vi "Add Tx Label.vi"(6 "transfer type":T2, 8 "error in":errorcluster, 9 "SDI value":T3=-1 items=["All"=-1, "0 (b00)"=0, "1 (b01)"=1, "2 (b10)"=2, "3 (b11)"=3], 10 "label value":u32, 11 "port ref":T1 format="%.0x") -> (0 "error out":errorcluster, 2 "label ref":T1 format="%.0x", 3 "port ref out":T1 format="%.0x")   [LabVIEW 2020, in "Ballard ARINC 429 Scripting.lvlib"]
uses:
  Ballard ARINC 429 Scripting.lvlib
  Shared/SDI.ctl
  Shared/Transfer Type.ctl
  <vilib>/NI VeriStand/Custom Device API/Custom Device Item Ref.ctl
  Shared/Label Properties.ctl
  Shared/Label.ctl
  <vilib>/NI VeriStand/Custom Device API/Custom Device Channel.ctl
  <vilib>/NI VeriStand/Custom Device API/Custom Device Channel Type.ctl
  Constants.vi
  <vilib>/NI VeriStand/Custom Device API/Custom Device API.lvlib
  ARINC 429/ARINC 429 Scripting.lvlib
  Import/ARINC 429 Import.lvlib
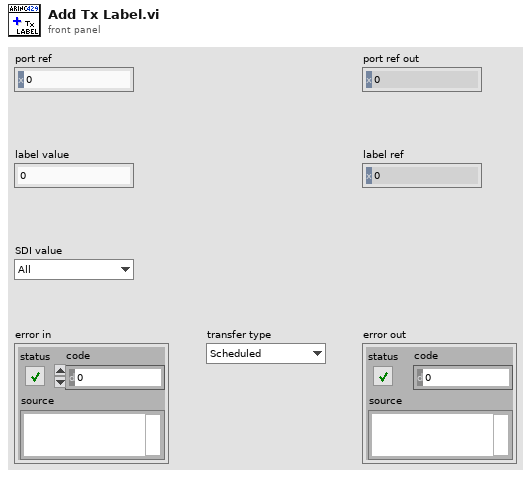
[diagram p1: front panel]
types:
  T1 = typedef "Custom Device API.lvlib/Custom Device Item Ref.ctl" = u64
  T2 = typedef "Transfer Type.ctl" = enum16{"Scheduled", "Acyclic", "Block", "Strobe"}
  T3 = typedef "SDI.ctl" = i32
  T4 = typedef "Direction.ctl" = enum16{"Rx", "Tx"}
  T5 = typedef "Custom Device API.lvlib/Custom Device Channel.ctl" = cluster{"Type":T6, "Units":string, "Default Value":dbl, "Faultable":bool, "Scalable":bool}
  T6 = typedef "Custom Device API.lvlib/Custom Device Channel Type.ctl" = enum16{"Input", "Output"}
  T7 = typedef "Label Properties.ctl" = cluster{"label (Dec)":T8, "SDI value":u8, "SDI enabled":bool}
  T8 = typedef "Label.ctl" = u8
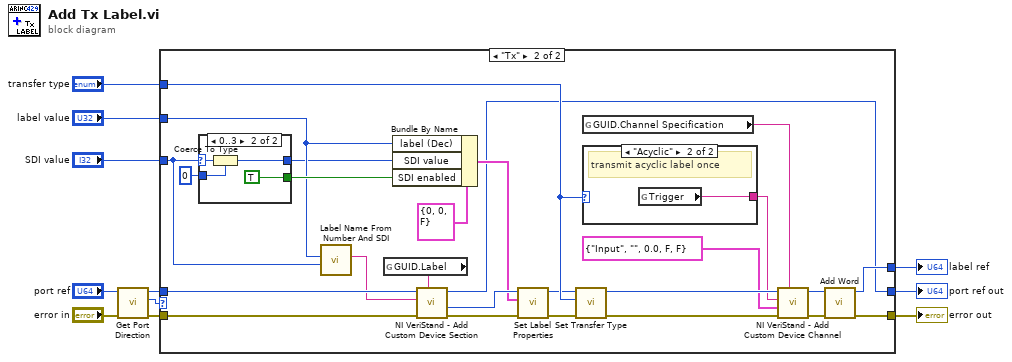
[diagram p0: block diagram]
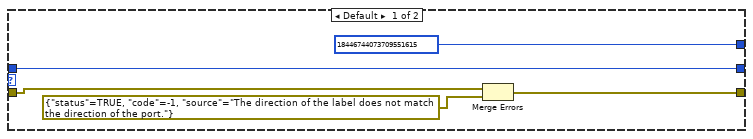
[diagram p2: hidden frame]
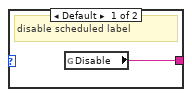
[diagram p3: hidden frame]
diagram:
  n1 = call "Get Port Direction.vi"("error in"="error in", "port ref in"="port ref") -> ("error out"=w7:errorcluster, "direction"=w1:T4, "port ref out"=w8:T1)  [unwired: 7 in]
  n2 = case shown="\"Tx\"" w1 {
    tunnel: [w13 w34] -> w11
    tunnel: w8 -> [w16 w31]
    tunnel: w7 -> [w14 w30]
    tunnel: [T1 18446744073709551615 ("label ref out") w27] -> w6
    tunnel: [w16 w17] -> w5
    tunnel: "transfer type" -> [_ w26]
    tunnel: "label value" -> [_ w23]
    tunnel: "SDI value" -> [_ w21]
    frame Default {
      n3 = Merge Errors(w14, errorcluster {"status"=TRUE, "code"=-1, "source"="The direction of the label does not match the direction of the port."} ("error in")) -> (w13:errorcluster)
    }
    frame "Tx" {
      n4 = case shown="0..3" w21 {
        selector: w21 -> [_ w49]
        tunnel: [w45 w46] -> w22
        tunnel: u8 0 ("SDI value") -> [w45 w48]
        tunnel: [_ TRUE] -> w28
        frame Default {
        }
        frame 0..3 {
          n5 = Coerce To Type(0:w49, 1:w48) -> (2:w46:u8)
        }
      }
      n6 = call "Label Name From Number And SDI.vi"("SDI value"=w21, "label (Dec)"=w23) -> ("label name"=w24:string)  [unwired: 9 in]
      n7 = global read "Constants.vi" "GUID.Label"() -> (w35:string)
      n8 = Bundle By Name(cluster=T7 {"label (Dec)"=0, "SDI value"=0, "SDI enabled"=FALSE} ("label properties"), "label (Dec)"=w23, "SDI value"=w22, "SDI enabled"=w28) -> (w32:T7)
      n9 = call <vilib>:"NI VeriStand - Add Custom Device Section.vi"("GUID (Default Section)"=w35, "error in (no error)"=w30, "Section Name"=w24, "Parent Ref in"=w31) -> ("error out"=w37:errorcluster, "Section Ptr"=w36:T1, "Parent Ref out"=w17:T1)  [unwired: 4 in, 1 out]
      n10 = call "Set Label Properties.vi"("error in"=w37, "label properties"=w32, "label ref"=w36) -> ("error out"=w38:errorcluster, "label ref out"=w25:T1)  [unwired: 7 in]
      n11 = call "Set Transfer Type.vi"("error in"=w38, "transfer type"=w26, "label ref in"=w25) -> ("error out"=w39:errorcluster, "label ref out"=w41:T1)  [unwired: 7 in]
      n12 = global read "Constants.vi" "GUID.Channel Specification"() -> (w20:string)
      n13 = case shown="\"Acyclic\"" w26 {
        tunnel: [w43 w44] -> w19
        frame Default {
          # "disable scheduled label"
          n14 = global read "Constants.vi" "Disable"() -> (w43:string)
        }
        frame "Acyclic" {
          # "transmit acyclic label once"
          n15 = global read "Constants.vi" "Trigger"() -> (w44:string)
        }
      }
      n16 = call <vilib>:"NI VeriStand - Add Custom Device Channel.vi"("GUID (Default Channel)"=w20, "error in (no error)"=w39, "Channel"=T5 {"Type"=enum."Input", "Units"="", "Default Value"=0.0, "Faultable"=FALSE, "Scalable"=FALSE}, "Channel Name"=w19, "Parent Ref in"=w41) -> ("error out"=w40:errorcluster, "Parent Ref out"=w42:T1)  [unwired: 3 in, 2 out]
      n17 = call "Add Word.vi"("error in"=w40, "label ref"=w42) -> ("error out"=w34:errorcluster, "label ref out"=w27:T1)  [unwired: 6 in, 2 out]
    }
  }
  "label ref" <- w6
  "error out" <- w11
  "port ref out" <- w5
